vi "DataManagementUpdateAnnotationIdRoutedMessage_Name.vi"() -> (1 "MessageName":string)   [LabVIEW 2017]
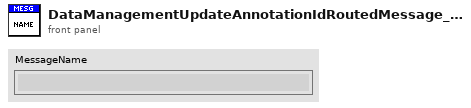
[diagram p1: front panel]
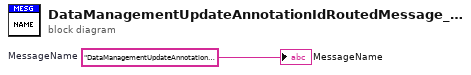
[diagram p0: block diagram]
diagram:
  w1 = "DataManagementUpdateAnnotationIdRoutedMessage"  # MessageName
  "MessageName" <- w1
